vi "Resiprocal.vi"() -> ()   [LabVIEW 2024]
panel:
  out "Numeric 2":dbl
  in  "Numeric":dbl
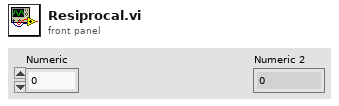
[diagram p1: front panel]
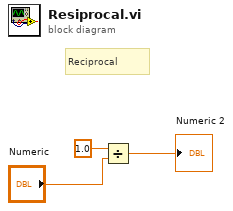
[diagram p0: block diagram]
diagram:
  # "Reciprocal"
  n1 = Divide(x=1.0, y="Numeric") -> (x/y=→"Numeric 2":dbl)
